vi "Get function range value frequency.vi"(8 "error in (no error)":errorcluster, 11 "VISA resource name":refnum<visa-resource-name>) -> (0 "error out":errorcluster, 1 "Value [?]":dbl, 2 "Frequency [Hz]":dbl, 3 "VISA resource name out":refnum<visa-resource-name>, 4 "Range code":i32, 5 "Fucntion code":i32, 6 "AC":bool, 7 "DC":bool)   [LabVIEW 2020, in "Datron D4xxx.lvlib"]
doc: "This VI returns range, value and frequency. In DC modes it returns zero frequency.s"
uses:
  Datron D4xxx.lvlib
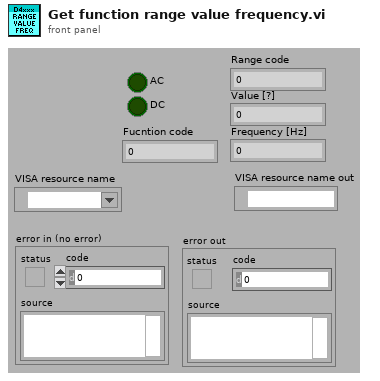
[diagram p1: front panel]
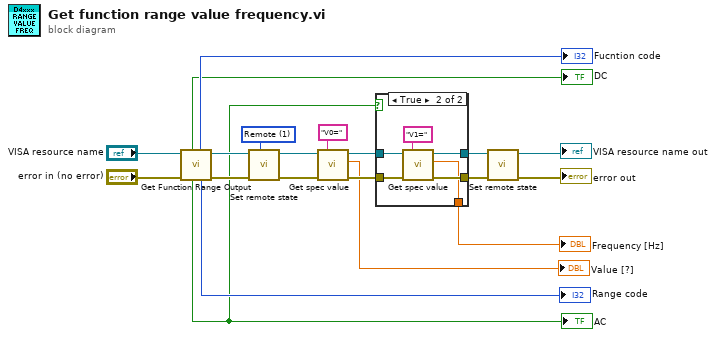
[diagram p0: block diagram]
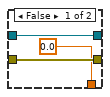
[diagram p2: hidden frame]
diagram:
  w14 = u16 1 items=["Local", "Remote", "Default"] ("Remote state")
  n1 = call "Get Function Range Output.vi"("error in (no error)"="error in (no error)", "VISA resource name"="VISA resource name") -> ("error out"=w19:errorcluster, "VISA resource name out"=w17:refnum<visa-resource-name>, "Range {R0-R9}"=→"Range code":i32, "Function {F0-F5}"=→"Fucntion code":i32, "AC"=w1:bool, "DC"=→"DC":bool)  [unwired: 2 in, 2 out]
  "AC" <- w1
  n2 = call "Set remote state.vi"("error in"=w19, "Remote state"=w14, "VISA resource name"=w17) -> ("error out"=w13:errorcluster, "VISA resource name out"=w12:refnum<visa-resource-name>)  [unwired: 7 in]
  n3 = call "Get spec value.vi"("error in (no error)"=w13, "Command string"="V0=", "VISA resource name"=w12) -> ("error out"=w10:errorcluster, "Value"=→"Value [?]":dbl, "VISA resource name out"=w8:refnum<visa-resource-name>)  [unwired: 5 in, 1 out]
  n4 = case shown="True" w1 {
    tunnel: w10 -> [w22 w28]
    tunnel: [w22 w27] -> w9
    tunnel: w8 -> [w23 w26]
    tunnel: [w23 w25] -> w7
    tunnel: [0.0 ("Value") w24] -> w6
    frame False {
    }
    frame True {
      n5 = call "Get spec value.vi"("error in (no error)"=w28, "Command string"="V1=", "VISA resource name"=w26) -> ("error out"=w27:errorcluster, "Value"=w24:dbl, "VISA resource name out"=w25:refnum<visa-resource-name>)  [unwired: 5 in, 1 out]
    }
  }
  "Frequency [Hz]" <- w6
  n6 = call "Set remote state.vi"("error in"=w9, "VISA resource name"=w7) -> ("error out"=→"error out":errorcluster, "VISA resource name out"=→"VISA resource name out":refnum<visa-resource-name>)  [unwired: 8 in]
